vi "newsubvi Robot GoTo XY.vi"(2 "GoToY":i32, 3 "GoToX":i32, 4 "Slow Speed":bool, 5 "VISA In":refnum<visa-resource-name>) -> (0 "error out":errorcluster, 1 "VISA Out":refnum<visa-resource-name>)   [LabVIEW 2012]
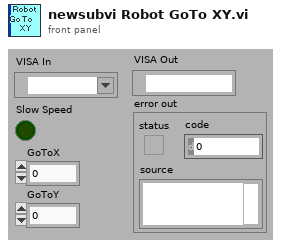
[diagram p1: front panel]
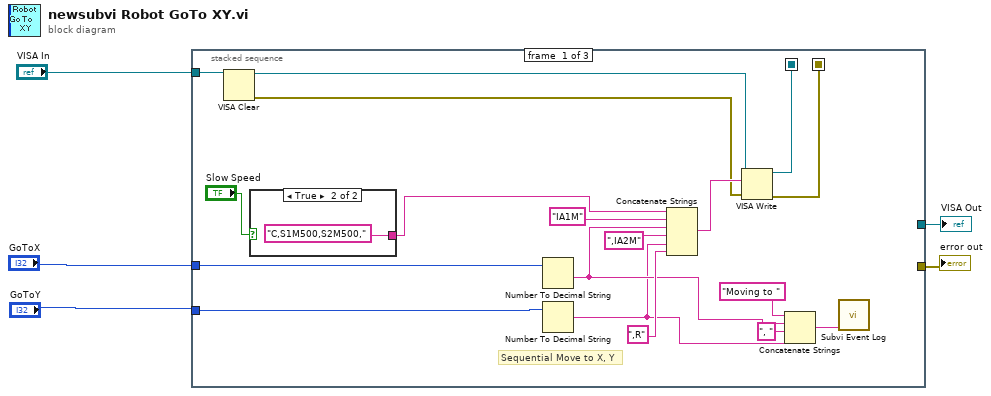
[diagram p0: block diagram]
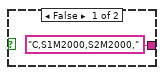
[diagram p2: hidden frame]
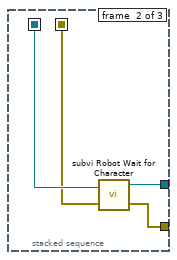
[diagram p3: hidden frame]
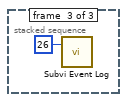
[diagram p4: hidden frame]
diagram:
  n1 = stacked-sequence {
    seq-local: [w7 _ _] -> [_ w29 _]
    seq-local: [w6 _ _] -> [_ w27 _]
    tunnel: "GoToY" -> [w18 _ _]
    tunnel: "GoToX" -> [w17 _ _]
    tunnel: "VISA In" -> [w11 _ _]
    tunnel: [_ w28 _] -> w2
    tunnel: [_ w26 _] -> w1
    frame #0 {
      # "Sequential Move to X, Y"
      n2 = VISA Clear(VISA resource name=w11) -> (VISA resource name out=w10:refnum<visa-resource-name>, error out=w8:errorcluster)  [unwired: 1 in]
      n3 = case shown="True" "Slow Speed" {
        tunnel: ["C,S1M2000,S2M2000," "C,S1M500,S2M500,"] -> w19
        frame False {
        }
        frame True {
        }
      }
      n4 = Number To Decimal String(number=w17) -> (decimal integer string=w15:string)  [unwired: 1 out]
      n5 = Number To Decimal String(number=w18) -> (decimal integer string=w13:string)  [unwired: 1 out]
      n6 = Concatenate Strings(w19, "IA1M" ("Text to Send"), w15, ",IA2M" ("Text to Send"), w13, ",R" ("Text to Send")) -> (w9:string)
      n7 = VISA Write(VISA resource name=w10, write buffer=w9, error in (no error)=w8) -> (VISA resource name out=w7:refnum<visa-resource-name>, error out=w6:errorcluster)  [unwired: 1 out]
      n8 = Concatenate Strings("Moving to " ("string"), w15, ", " ("string"), w13) -> (w12:string)
      n9 = call "Subvi Event Log.vi"("CustomMessage"=w12) -> ()  [unwired: 1 in]
    }
    frame #1 {
      n10 = call "subvi Robot Wait for Character.vi"("error in"=w27, "VISA In"=w29) -> ("error out"=w26:errorcluster, "VISA Out"=w28:refnum<visa-resource-name>)
    }
    frame #2 {
      n11 = call "Subvi Event Log.vi"("EventNum"=u32 26) -> ()  [unwired: 1 in]
    }
  }
  "error out" <- w1
  "VISA Out" <- w2
